vi "Autonomous Independent.vi"   [LabVIEW 2016]
doc: "This VI is called when autonomous begins, and will automatically be terminated when autonomous ends. You can carry out timed or sensor driven robot movement independently without needing to return to the caller."
uses:
  <vilib>/Rock Robotics/WPI/Solenoid/WPI_SolenoidValue.ctl
  <vilib>/Rock Robotics/WPI/Utilities/WPI_GetSetVariantRefNum.vi
  <vilib>/Rock Robotics/Network Tables/NT Read String.vi
  <vilib>/Rock Robotics/Network Tables/NT Write Numeric Array.vi
  Robot Global Data.vi
  <vilib>/Rock Robotics/WPI/Solenoid/WPI_SolenoidSetEnum.vi
  <vilib>/addons/control/pid/pid.llb/PID (DBL).vi
  <vilib>/addons/control/pid/NI_PID_pid.lvlib
panel:
  # "Be sure to right-click and choose Data Operations>>Make Current Value default if you want to save the array values with the VI"
types:
  T1 = typedef "WPI_JoystickDevRef.ctl" = cluster{"Device":T2}
  T2 = typedef "WPI_JoystickDeviceEnum.ctl" = enum16{"USB 0", "USB 1", "USB 2", "USB 3", "USB 4", "USB 5"}
  T3 = typedef "WPI_RobotDriveDevRef.ctl" = cluster{"DevStatus":errorcluster, "Motors[]":T4[], "Square Inputs":bool, "Max Output":dbl}
  T4 = typedef "WPI_MotorControlDeviceRef.ctl" = cluster{"DeviceStatus":errorcluster, "Type":T5, "PWM":cluster{"PWM Channel":T6, "DeadBand":T7}, "CAN":cluster{"Device Number":u8, "SetOutput VI Ref":variant, "GetOutput VI Ref":variant, "Enable VI Ref":variant, "Disable VI Ref":variant, "Data":variant}, "Invert":bool}
  T5 = typedef "WPI_MotorControlType.ctl" = enum16{"PWM", "CAN"}
  T6 = typedef "FPGA_DIOPWMChannel.ctl" = enum8{"PWM 0", "PWM 1", "PWM 2", "PWM 3", "PWM 4", "PWM 5", "PWM 6", "PWM 7", "PWM 8", "PWM 9", "PWM MXP 0", "PWM MXP 1", "PWM MXP 2", "PWM MXP 3", "PWM MXP 4", "PWM MXP 5", "PWM MXP 6", "PWM MXP 7", "PWM MXP 8", "PWM MXP 9", "Invalid"}
  T7 = typedef "WPI_PWMDeadband.ctl" = cluster{"Name":string, "maxPositivePwm":i32, "minPositivePwm":i32, "centerPwm":i32, "maxNegativePwm":i32, "minNegativePwm":i32, "angularRange":u16}
  T8 = typedef "WPI_EncoderDevRef.ctl" = cluster{"DevStatus":errorcluster, "EncoderIndex":T9, "CounterIndex":T10, "DistancePerCount":dbl, "Decoding Type":T11}
  T9 = typedef "FPGA_EncoderIdx.ctl" = enum8{"Enc 0", "Enc 1", "Enc 2", "Enc 3", "Enc 4", "Enc 5", "Enc 6", "Enc 7", "Invalid"}
  T10 = typedef "FPGA_CounterCtrSystemIndex.ctl" = enum8{"Ctr 0", "Ctr 1", "Ctr 2", "Ctr 3", "Ctr 4", "Ctr 5", "Ctr 6", "Ctr 7", "Invalid"}
  T11 = typedef "WPI_EncoderType.ctl" = enum16{"1x", "2x", "4x"}
  T12 = typedef "WPI_SolenoidDevRef.ctl" = cluster{"DevStatus":errorcluster, "Pneumatics Control Module":u8, "Forward Solenoid Channel":T13, "Reverse Solenoid Channel":T13}
  T13 = typedef "WPI_SolenoidChannel.ctl" = enum8{"Solenoid 0", "Solenoid 1", "Solenoid 2", "Solenoid 3", "Solenoid 4", "Solenoid 5", "Solenoid 6", "Solenoid 7", "Invalid"}
  T14 = typedef "WPI_SolenoidValue.ctl" = enum16{"Off", "On", "Forward", "Reverse"}
  T15 = cluster{"proportional gain (Kc)":dbl, "integral time (Ti, min)":dbl, "derivative time (Td, min)":dbl}
  T16 = cluster{"Yaw":dbl, "Roll":dbl, "Pitch":dbl, "Heading":dbl, "Fused Heading":dbl}
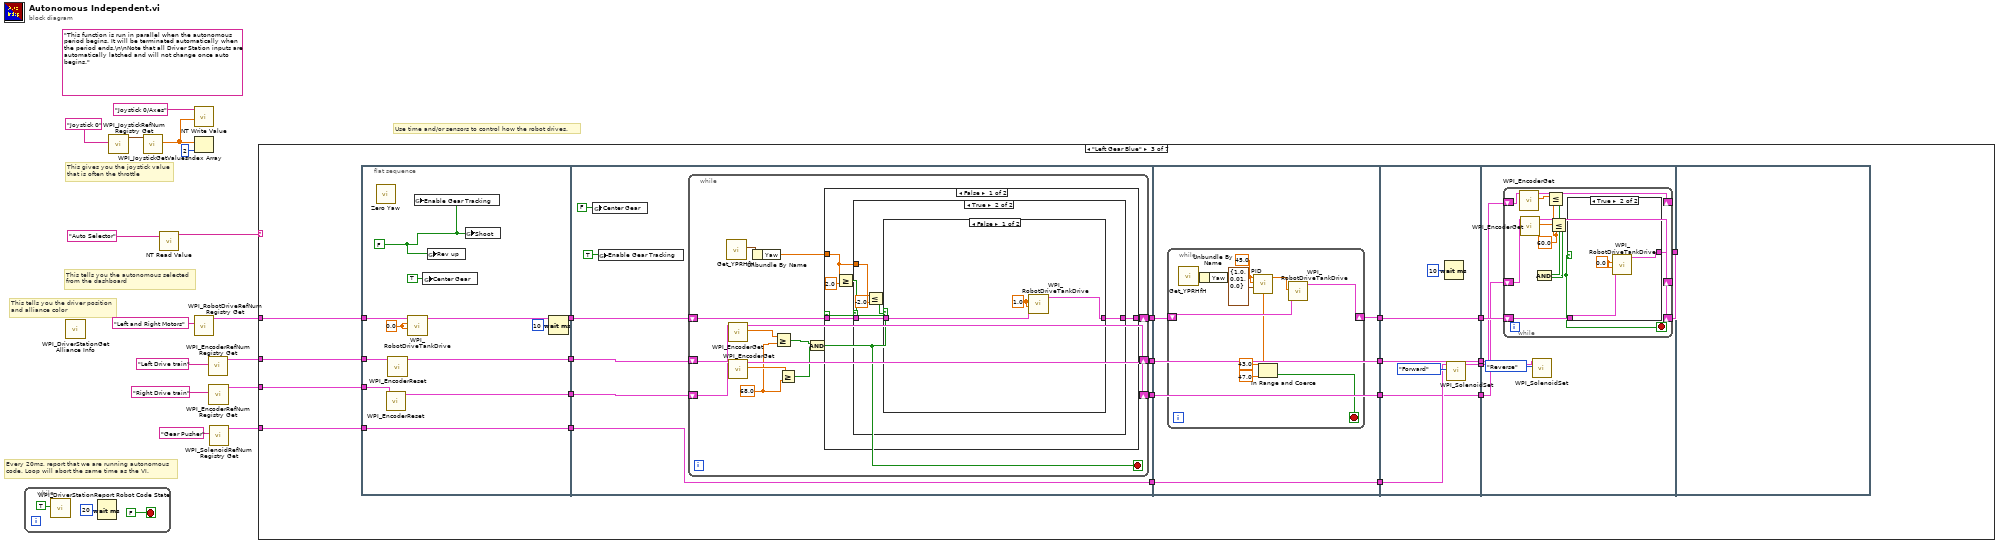
[diagram p0: block diagram]
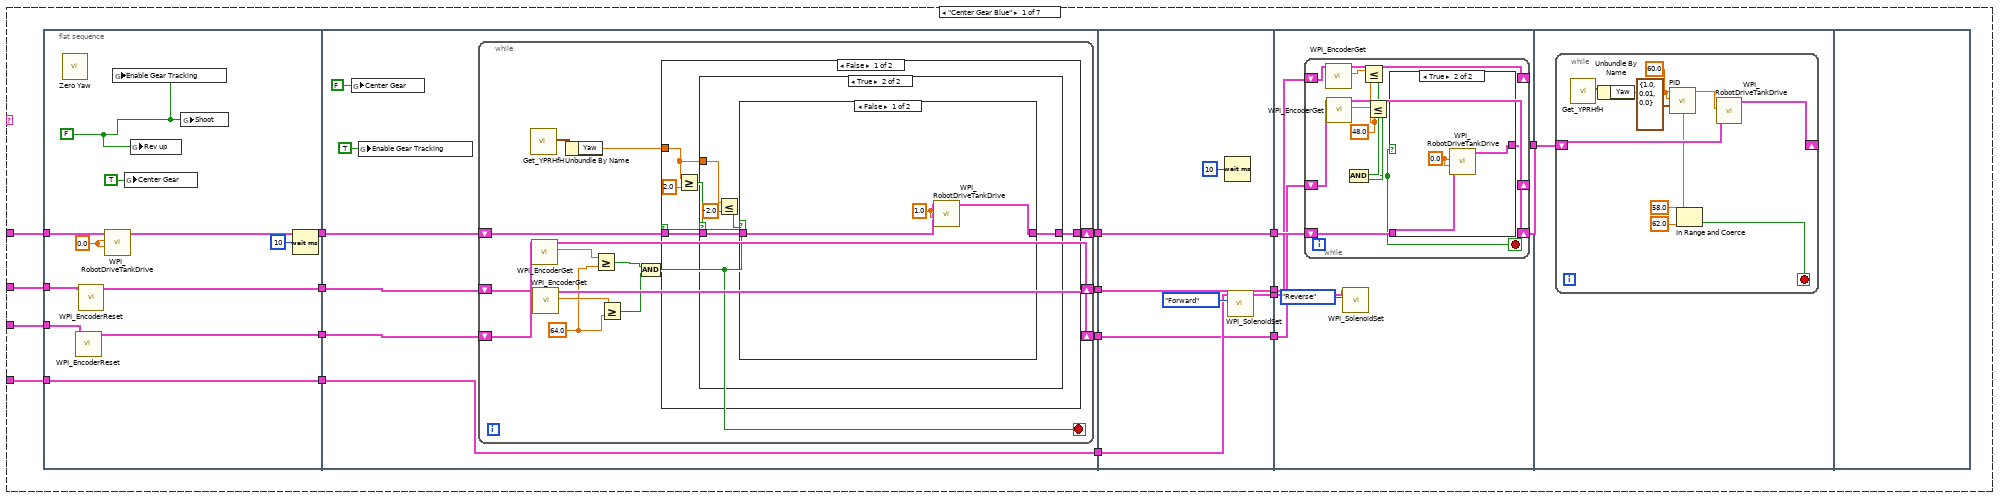
[diagram p2: hidden frame]
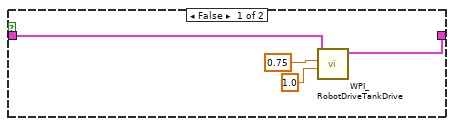
[diagram p3: hidden frame]
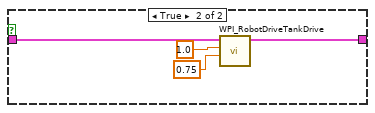
[diagram p4: hidden frame]
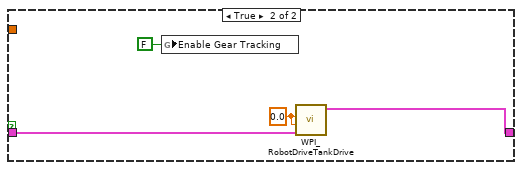
[diagram p5: hidden frame]
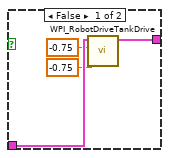
[diagram p6: hidden frame]
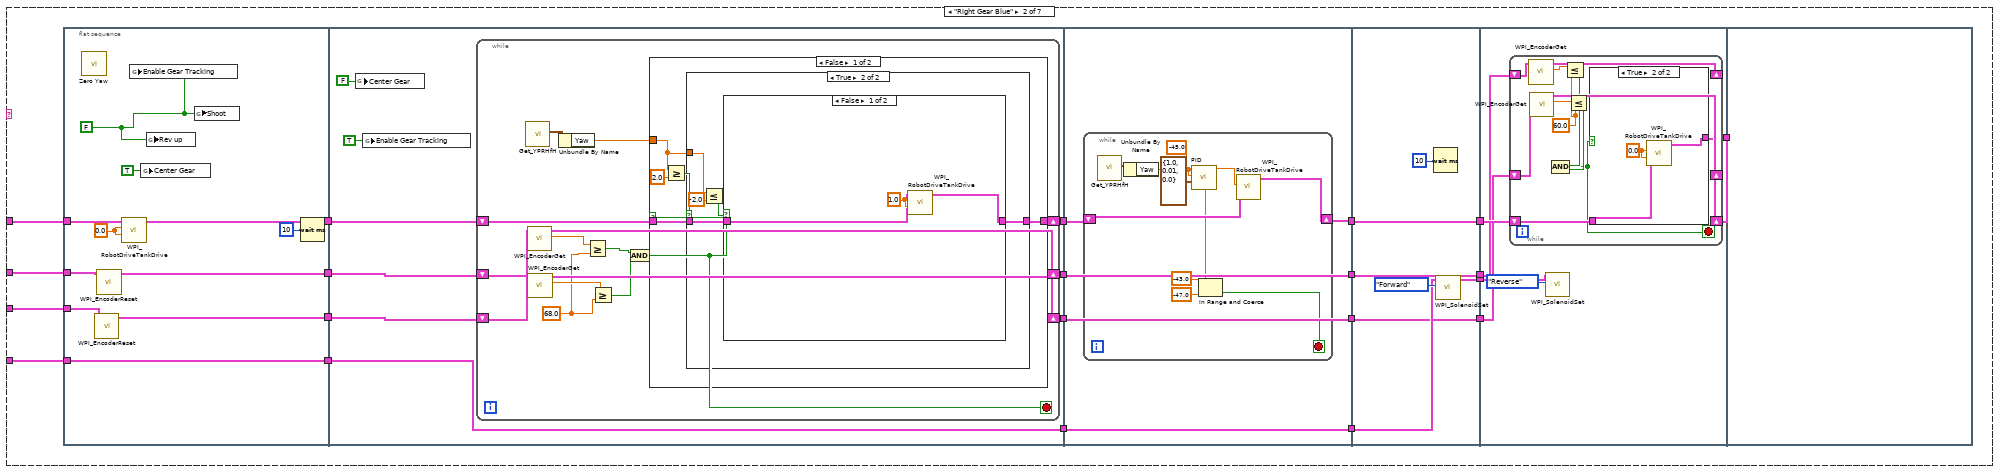
[diagram p7: hidden frame]
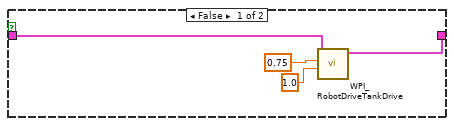
[diagram p8: hidden frame]
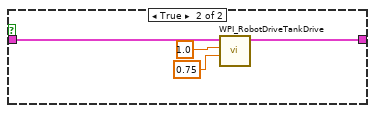
[diagram p9: hidden frame]
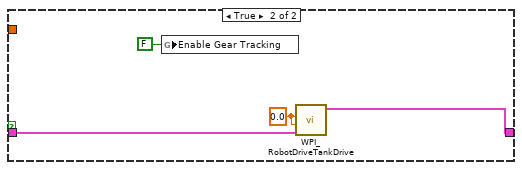
[diagram p10: hidden frame]
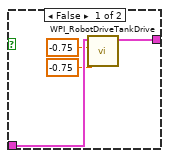
[diagram p11: hidden frame]
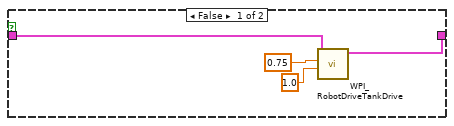
[diagram p12: hidden frame]
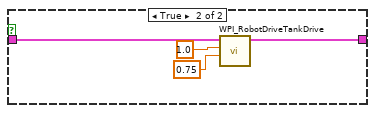
[diagram p13: hidden frame]
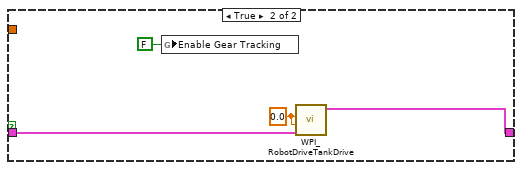
[diagram p14: hidden frame]
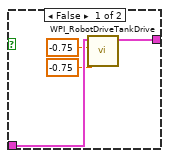
[diagram p15: hidden frame]
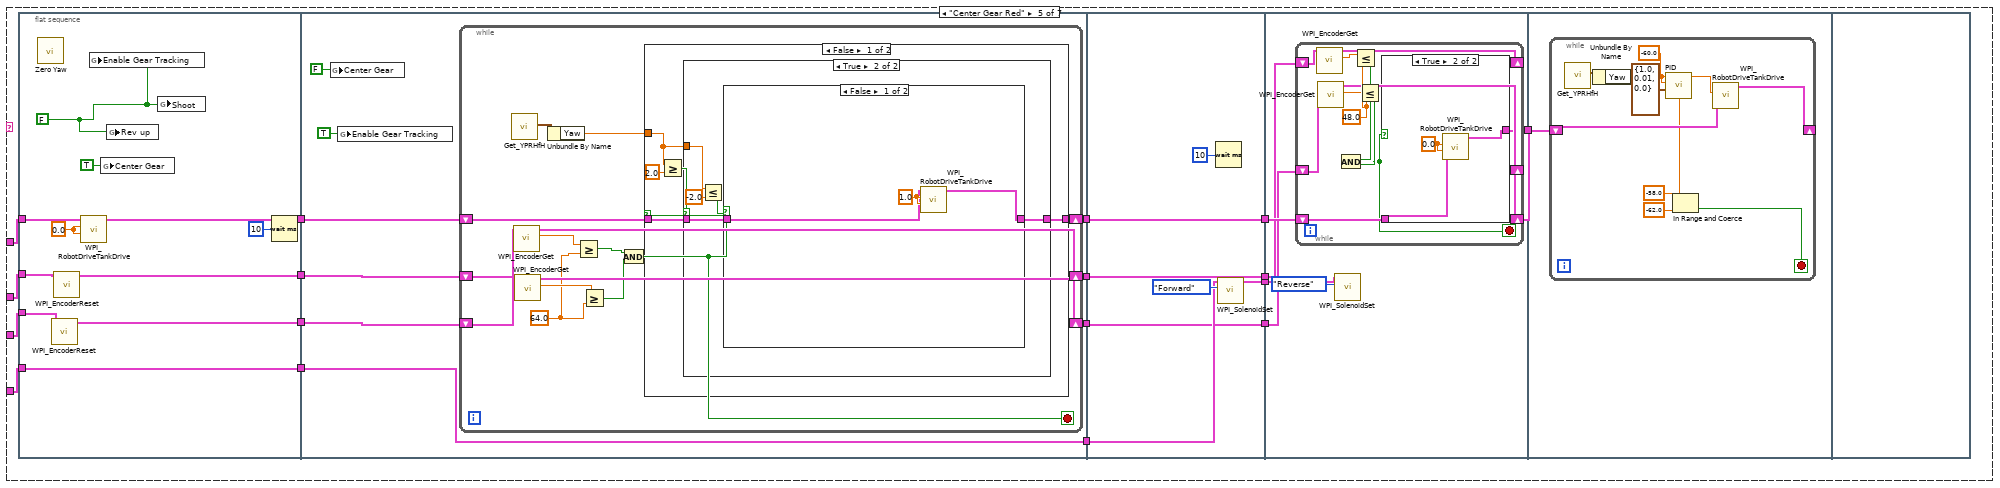
[diagram p17: hidden frame]
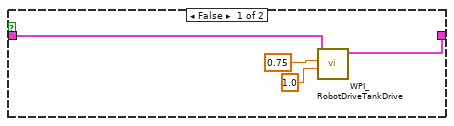
[diagram p18: hidden frame]
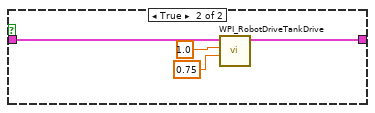
[diagram p19: hidden frame]
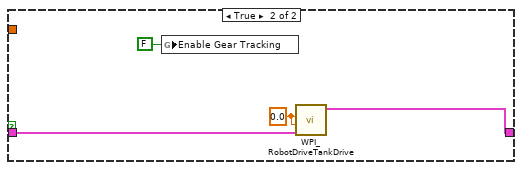
[diagram p20: hidden frame]
diagram:
  (unwired) "This function is run in parallel when the autonomous period begins. It will be terminated automatically when the period ends.\n\nNote that all Driver Station inputs are automatically latched and will not change once auto begins."
  # "This tells you the autonomous selected\nfrom the dashboard"
  # "Every 20ms, report that we are running autonomous\ncode. Loop will abort the same time as the VI."
  # "This gives you the joystick value\nthat is often the throttle"
  # "Use time and/or sensors to control how the robot drives."
  # "This tells you the driver position\nand alliance color"
  n1 = while {
    stop <- FALSE stop-if-true
    n2 = call <vilib>:"WPI_DriverStationReport Robot Code State.vi"("Autonomous"=TRUE) -> ()  [unwired: 10 in, 1 out]
    n3 = Wait (ms)(milliseconds to wait=u32 20) -> ()  [unwired: 1 out]
  }
  n4 = call <vilib>:"WPI_DriverStationGet Alliance Info.vi"() -> ()  [unwired: 12 out]
  n5 = call <vilib>:"WPI_JoystickRefNum Registry Get.vi"("refnum name"="Joystick 0") -> ("JoystickDevRef"=w14:T1)  [unwired: 1 in, 9 out]
  n6 = call <vilib>:"WPI_JoystickGetValues.vi"("JoystickDevRef"=w14) -> ("Axes"=w10:dbl[])  [unwired: 6 in, 4 out]
  n7 = call-poly <vilib>:"NT Read Value.vi"("Name"="Auto Selector") -> ("String"=w11:string)  [unwired: 9 in, 1 out]
  n8 = call-poly <vilib>:"NT Write Value.vi"("Numeric Array"=w10, "Name"="Joystick 0/Axes") -> ()  [unwired: 9 in, 1 out]
  n9 = Index Array(array=w10, index=2) -> ()  [unwired: 1 out]
  n10 = call <vilib>:"WPI_RobotDriveRefNum Registry Get.vi"("refnum name"="Left and Right Motors") -> ("RobotDriveDevRef"=w7:T3)  [unwired: 9 in, 1 out]
  n11 = call <vilib>:"WPI_EncoderRefNum Registry Get.vi"("refnum name"="Left Drive train") -> ("EncoderDevRef"=w4:T8)  [unwired: 9 in, 1 out]
  n12 = call <vilib>:"WPI_EncoderRefNum Registry Get.vi"("refnum name"="Right Drive train") -> ("EncoderDevRef"=w3:T8)  [unwired: 9 in, 1 out]
  n13 = call <vilib>:"WPI_SolenoidRefNum Registry Get.vi"("refnum name"="Gear Pusher") -> ("SolenoidDevRef"=w1:T12)  [unwired: 9 in, 1 out]
  n14 = case shown="\"Left Gear Blue\"" w11 {
    tunnel: w7 -> [w22 w138 w268 _ w408 w519 w641]
    tunnel: w4 -> [w21 w139 w267 _ w407 w520 w640]
    tunnel: w3 -> [w20 w140 w266 _ w406 w521 w639]
    tunnel: w1 -> [w19 w141 w265 _ w400 w522 w638]
    frame "Center Gear Blue" {
      n15 = flat-sequence {
        tunnel: w22 -> [w45]
        tunnel: w21 -> [w44]
        tunnel: w20 -> [w43]
        tunnel: [w39] -> w35
        tunnel: [w38] -> w34
        tunnel: [w37] -> w33
        tunnel: [w36] -> w32
        tunnel: w19 -> [w36]
        tunnel: w35 -> [w55]
        tunnel: w34 -> [w54]
        tunnel: w33 -> [w51]
        tunnel: [w50] -> w31
        tunnel: w32 -> [w50]
        tunnel: [w49] -> w30
        tunnel: [w48] -> w29
        tunnel: [w47] -> w28
        tunnel: w31 -> [w100]
        tunnel: [w98] -> w27
        tunnel: [w97] -> w26
        tunnel: w30 -> [w97]
        tunnel: [w96] -> w25
        tunnel: w29 -> [w96]
        tunnel: [w95] -> w24
        tunnel: w28 -> [w95]
        tunnel: w27 -> [w106]
        tunnel: w26 -> [w105]
        tunnel: w25 -> [w103]
        tunnel: w24 -> [w104]
        tunnel: [w102] -> w23
        tunnel: w23 -> [w127]
        frame #0 {
          w42 = FALSE
          w46 = 0.0 ("Left axis value")
          n16 = call <vilib>:"Zero Yaw.vi"() -> ()  [unwired: 12 in]
          n17 = call <vilib>:"WPI_EncoderReset.vi"("EncoderDevRef"=w43) -> ("EncoderDevRef"=w38:T8)  [unwired: 9 in, 1 out]
          n18 = call <vilib>:"WPI_EncoderReset.vi"("EncoderDevRef"=w44) -> ("EncoderDevRef"=w39:T8)  [unwired: 9 in, 1 out]
          n19 = call <vilib>:"WPI_RobotDriveTankDrive.vi"("Right axis value"=w46, "Left axis value"=w46, "RobotDriveDevRef"=w45) -> ("RobotDriveDevRef"=w37:T3)  [unwired: 6 in, 2 out]
          n20 = global write "Robot Global Data.vi" "Enable Gear Tracking"(w42) -> ()
          n21 = global write "Robot Global Data.vi" "Center Gear"(TRUE ("Center Gear")) -> ()
          n22 = global write "Robot Global Data.vi" "Rev up"(w42) -> ()
          n23 = global write "Robot Global Data.vi" "Shoot"(w42) -> ()
          n24 = Wait (ms)(milliseconds to wait=u32 10) -> ()  [unwired: 1 out]
        }
        frame #1 {
          n25 = global write "Robot Global Data.vi" "Center Gear"(FALSE ("Center Gear")) -> ()
          n26 = global write "Robot Global Data.vi" "Enable Gear Tracking"(TRUE ("Enable Gear Tracking")) -> ()
          n27 = while {
            shift-right: [w67] -> w48
            shift-left: w55 -> [w69]
            shift-right: [w66] -> w47
            shift-left: w54 -> [w68]
            shift-right: [w59] -> w49
            shift-left: w51 -> [w60]
            stop <- w63 stop-if-true
            w57 = 64.0
            n28 = call <vilib>:"Get_YPRHfH.vi"() -> ("YRPHfH"=w62:T16)  [unwired: 11 in]
            n29 = call <vilib>:"WPI_EncoderGet.vi"("EncoderDevRef"=w69) -> ("Distance"=w58:dbl, "EncoderDevRef"=w67:T8)  [unwired: 5 in, 4 out]
            n30 = call <vilib>:"WPI_EncoderGet.vi"("EncoderDevRef"=w68) -> ("Distance"=w65:dbl, "EncoderDevRef"=w66:T8)  [unwired: 5 in, 4 out]
            n31 = Unbundle By Name(w62) -> ("Yaw"=w61:dbl)
            n32 = Greater Or Equal?(x=w58, y=w57) -> (x >= y?=w56:bool)
            n33 = Greater Or Equal?(x=w65, y=w57) -> (x >= y?=w64:bool)
            n34 = Compound Arithmetic op=AND(w56, w64) -> (w63:bool)
            n35 = case shown="False" w63 {
              tunnel: w61 -> [w72 _]
              tunnel: w60 -> [w71 w93]
              tunnel: [w70 w92] -> w59
              frame False {
                n36 = Greater Or Equal?(x=w72, y=2.0) -> (x >= y?=w73:bool)
                n37 = case shown="True" w73 {
                  tunnel: w72 -> [_ w83]
                  tunnel: w71 -> [w76 w80]
                  tunnel: [w75 w79] -> w70
                  frame False {
                    n38 = call <vilib>:"WPI_RobotDriveTankDrive.vi"("Right axis value"=1.0, "Left axis value"=0.75, "RobotDriveDevRef"=w76) -> ("RobotDriveDevRef"=w75:T3)  [unwired: 6 in, 2 out]
                  }
                  frame True {
                    n39 = Less Or Equal?(x=w83, y=-2.0) -> (x <= y?=w81:bool)
                    n40 = case shown="False" w81 {
                      tunnel: w80 -> [w85 w88]
                      tunnel: [w84 w87] -> w79
                      frame False {
                        w86 = 1.0 ("Left axis value")
                        n41 = call <vilib>:"WPI_RobotDriveTankDrive.vi"("Right axis value"=w86, "Left axis value"=w86, "RobotDriveDevRef"=w85) -> ("RobotDriveDevRef"=w84:T3)  [unwired: 6 in, 2 out]
                      }
                      frame True {
                        n42 = call <vilib>:"WPI_RobotDriveTankDrive.vi"("Right axis value"=0.75, "Left axis value"=1.0, "RobotDriveDevRef"=w88) -> ("RobotDriveDevRef"=w87:T3)  [unwired: 6 in, 2 out]
                      }
                    }
                  }
                }
              }
              frame True {
                w94 = 0.0 ("Left axis value")
                n43 = global write "Robot Global Data.vi" "Enable Gear Tracking"(FALSE ("Enable Gear Tracking")) -> ()
                n44 = call <vilib>:"WPI_RobotDriveTankDrive.vi"("Right axis value"=w94, "Left axis value"=w94, "RobotDriveDevRef"=w93) -> ("RobotDriveDevRef"=w92:T3)  [unwired: 6 in, 2 out]
              }
            }
          }
        }
        frame #2 {
          n45 = Wait (ms)(milliseconds to wait=u32 10) -> ()  [unwired: 1 out]
          n46 = call-poly <vilib>:"WPI_SolenoidSet.vi"("Value"=WPI_SolenoidValue."Forward", "SolenoidDevRef"=w100) -> ("SolenoidDevRef"=w98:T12)  [unwired: 8 in, 1 out]
        }
        frame #3 {
          n47 = while {
            shift-right: [w112] -> _
            shift-left: w104 -> [w114]
            shift-right: [w113] -> _
            shift-left: w103 -> [w115]
            shift-right: [w108] -> w102
            shift-left: w105 -> [w119]
            stop <- w109 stop-if-true
            w117 = 48.0
            n48 = call <vilib>:"WPI_EncoderGet.vi"("EncoderDevRef"=w115) -> ("Distance"=w118:dbl, "EncoderDevRef"=w113:T8)  [unwired: 5 in, 4 out]
            n49 = call <vilib>:"WPI_EncoderGet.vi"("EncoderDevRef"=w114) -> ("Distance"=w116:dbl, "EncoderDevRef"=w112:T8)  [unwired: 5 in, 4 out]
            n50 = Less Or Equal?(x=w118, y=w117) -> (x <= y?=w111:bool)
            n51 = Less Or Equal?(x=w116, y=w117) -> (x <= y?=w110:bool)
            n52 = Compound Arithmetic op=AND(w111, w110) -> (w109:bool)
            n53 = case shown="True" w109 {
              tunnel: w119 -> [w123 w125]
              tunnel: [w120 w124] -> w108
              frame False {
                n54 = call <vilib>:"WPI_RobotDriveTankDrive.vi"("Right axis value"=-0.75, "Left axis value"=-0.75, "RobotDriveDevRef"=w123) -> ("RobotDriveDevRef"=w120:T3)  [unwired: 6 in, 2 out]
              }
              frame True {
                w126 = 0.0 ("Left axis value")
                n55 = call <vilib>:"WPI_RobotDriveTankDrive.vi"("Right axis value"=w126, "Left axis value"=w126, "RobotDriveDevRef"=w125) -> ("RobotDriveDevRef"=w124:T3)  [unwired: 6 in, 2 out]
              }
            }
          }
          n56 = call-poly <vilib>:"WPI_SolenoidSet.vi"("Value"=WPI_SolenoidValue."Reverse", "SolenoidDevRef"=w106) -> ()  [unwired: 8 in, 2 out]
        }
        frame #4 {
          n57 = while {
            shift-right: [w132] -> _
            shift-left: w127 -> [w133]
            stop <- w128 stop-if-true
            n58 = call <vilib>:"Get_YPRHfH.vi"() -> ("YRPHfH"=w137:T16)  [unwired: 11 in]
            n59 = Unbundle By Name(w137) -> ("Yaw"=w131:dbl)
            n60 = call-poly <vilib>:"PID.vi"("PID gains"=T15 {"proportional gain (Kc)"=1.0, "integral time (Ti, min)"=0.01, "derivative time (Td, min)"=0.0}, "process variable"=w131, "setpoint"=60.0) -> ("output"=w134:dbl)  [unwired: 7 in, 1 out]
            n61 = In Range and Coerce(upper limit=58.0, x=w131, lower limit=62.0) -> (In Range?=w128:bool)  [unwired: 1 out]
            n62 = call <vilib>:"WPI_RobotDriveTankDrive.vi"("Left axis value"=w134, "RobotDriveDevRef"=w133) -> ("RobotDriveDevRef"=w132:T3)  [unwired: 7 in, 2 out]
          }
        }
        frame #5 {
        }
      }
    }
    frame "Right Gear Blue" {
      n63 = flat-sequence {
        tunnel: w138 -> [w168]
        tunnel: w139 -> [w167]
        tunnel: [w163] -> w158
        tunnel: [w162] -> w157
        tunnel: [w161] -> w156
        tunnel: [w160] -> w155
        tunnel: w141 -> [w160]
        tunnel: w140 -> [w159]
        tunnel: w158 -> [w178]
        tunnel: w157 -> [w177]
        tunnel: w156 -> [w174]
        tunnel: [w173] -> w154
        tunnel: w155 -> [w173]
        tunnel: [w172] -> w153
        tunnel: [w171] -> w152
        tunnel: [w170] -> w151
        tunnel: w154 -> [w222]
        tunnel: [w222] -> w150
        tunnel: w153 -> [w221]
        tunnel: [w220] -> w149
        tunnel: w152 -> [w219]
        tunnel: [w219] -> w148
        tunnel: w151 -> [w218]
        tunnel: [w218] -> w147
        tunnel: w150 -> [w238]
        tunnel: [w236] -> w146
        tunnel: [w235] -> w145
        tunnel: w149 -> [w235]
        tunnel: [w234] -> w144
        tunnel: w148 -> [w234]
        tunnel: [w233] -> w143
        tunnel: w147 -> [w233]
        tunnel: w146 -> [w244]
        tunnel: w145 -> [w243]
        tunnel: w144 -> [w241]
        tunnel: w143 -> [w242]
        tunnel: [w240] -> w142
        tunnel: w142 -> [_]
        frame #0 {
          w166 = FALSE
          w169 = 0.0 ("Left axis value")
          n64 = call <vilib>:"Zero Yaw.vi"() -> ()  [unwired: 12 in]
          n65 = call <vilib>:"WPI_EncoderReset.vi"("EncoderDevRef"=w159) -> ("EncoderDevRef"=w162:T8)  [unwired: 9 in, 1 out]
          n66 = call <vilib>:"WPI_EncoderReset.vi"("EncoderDevRef"=w167) -> ("EncoderDevRef"=w163:T8)  [unwired: 9 in, 1 out]
          n67 = call <vilib>:"WPI_RobotDriveTankDrive.vi"("Right axis value"=w169, "Left axis value"=w169, "RobotDriveDevRef"=w168) -> ("RobotDriveDevRef"=w161:T3)  [unwired: 6 in, 2 out]
          n68 = global write "Robot Global Data.vi" "Enable Gear Tracking"(w166) -> ()
          n69 = global write "Robot Global Data.vi" "Center Gear"(TRUE ("Center Gear")) -> ()
          n70 = global write "Robot Global Data.vi" "Rev up"(w166) -> ()
          n71 = global write "Robot Global Data.vi" "Shoot"(w166) -> ()
          n72 = Wait (ms)(milliseconds to wait=u32 10) -> ()  [unwired: 1 out]
        }
        frame #1 {
          n73 = global write "Robot Global Data.vi" "Center Gear"(FALSE ("Center Gear")) -> ()
          n74 = global write "Robot Global Data.vi" "Enable Gear Tracking"(TRUE ("Enable Gear Tracking")) -> ()
          n75 = while {
            shift-right: [w190] -> w171
            shift-left: w178 -> [w192]
            shift-right: [w189] -> w170
            shift-left: w177 -> [w191]
            shift-right: [w182] -> w172
            shift-left: w174 -> [w183]
            stop <- w186 stop-if-true
            w180 = 68.0
            n76 = call <vilib>:"Get_YPRHfH.vi"() -> ("YRPHfH"=w185:T16)  [unwired: 11 in]
            n77 = call <vilib>:"WPI_EncoderGet.vi"("EncoderDevRef"=w192) -> ("Distance"=w181:dbl, "EncoderDevRef"=w190:T8)  [unwired: 5 in, 4 out]
            n78 = call <vilib>:"WPI_EncoderGet.vi"("EncoderDevRef"=w191) -> ("Distance"=w188:dbl, "EncoderDevRef"=w189:T8)  [unwired: 5 in, 4 out]
            n79 = Unbundle By Name(w185) -> ("Yaw"=w184:dbl)
            n80 = Greater Or Equal?(x=w181, y=w180) -> (x >= y?=w179:bool)
            n81 = Greater Or Equal?(x=w188, y=w180) -> (x >= y?=w187:bool)
            n82 = Compound Arithmetic op=AND(w179, w187) -> (w186:bool)
            n83 = case shown="False" w186 {
              tunnel: w184 -> [w195 _]
              tunnel: w183 -> [w194 w216]
              tunnel: [w193 w215] -> w182
              frame False {
                n84 = Greater Or Equal?(x=w195, y=2.0) -> (x >= y?=w196:bool)
                n85 = case shown="True" w196 {
                  tunnel: w195 -> [_ w206]
                  tunnel: w194 -> [w199 w203]
                  tunnel: [w198 w202] -> w193
                  frame False {
                    n86 = call <vilib>:"WPI_RobotDriveTankDrive.vi"("Right axis value"=1.0, "Left axis value"=0.75, "RobotDriveDevRef"=w199) -> ("RobotDriveDevRef"=w198:T3)  [unwired: 6 in, 2 out]
                  }
                  frame True {
                    n87 = Less Or Equal?(x=w206, y=-2.0) -> (x <= y?=w204:bool)
                    n88 = case shown="False" w204 {
                      tunnel: w203 -> [w208 w211]
                      tunnel: [w207 w210] -> w202
                      frame False {
                        w209 = 1.0 ("Left axis value")
                        n89 = call <vilib>:"WPI_RobotDriveTankDrive.vi"("Right axis value"=w209, "Left axis value"=w209, "RobotDriveDevRef"=w208) -> ("RobotDriveDevRef"=w207:T3)  [unwired: 6 in, 2 out]
                      }
                      frame True {
                        n90 = call <vilib>:"WPI_RobotDriveTankDrive.vi"("Right axis value"=0.75, "Left axis value"=1.0, "RobotDriveDevRef"=w211) -> ("RobotDriveDevRef"=w210:T3)  [unwired: 6 in, 2 out]
                      }
                    }
                  }
                }
              }
              frame True {
                w217 = 0.0 ("Left axis value")
                n91 = global write "Robot Global Data.vi" "Enable Gear Tracking"(FALSE ("Enable Gear Tracking")) -> ()
                n92 = call <vilib>:"WPI_RobotDriveTankDrive.vi"("Right axis value"=w217, "Left axis value"=w217, "RobotDriveDevRef"=w216) -> ("RobotDriveDevRef"=w215:T3)  [unwired: 6 in, 2 out]
              }
            }
          }
        }
        frame #2 {
          n93 = while {
            shift-right: [w227] -> w220
            shift-left: w221 -> [w228]
            stop <- w223 stop-if-true
            n94 = call <vilib>:"Get_YPRHfH.vi"() -> ("YRPHfH"=w232:T16)  [unwired: 11 in]
            n95 = Unbundle By Name(w232) -> ("Yaw"=w226:dbl)
            n96 = call-poly <vilib>:"PID.vi"("PID gains"=T15 {"proportional gain (Kc)"=1.0, "integral time (Ti, min)"=0.01, "derivative time (Td, min)"=0.0}, "process variable"=w226, "setpoint"=-45.0) -> ("output"=w229:dbl)  [unwired: 7 in, 1 out]
            n97 = In Range and Coerce(upper limit=-43.0, x=w226, lower limit=-47.0) -> (In Range?=w223:bool)  [unwired: 1 out]
            n98 = call <vilib>:"WPI_RobotDriveTankDrive.vi"("Left axis value"=w229, "RobotDriveDevRef"=w228) -> ("RobotDriveDevRef"=w227:T3)  [unwired: 7 in, 2 out]
          }
        }
        frame #3 {
          n99 = Wait (ms)(milliseconds to wait=u32 10) -> ()  [unwired: 1 out]
          n100 = call-poly <vilib>:"WPI_SolenoidSet.vi"("Value"=WPI_SolenoidValue."Forward", "SolenoidDevRef"=w238) -> ("SolenoidDevRef"=w236:T12)  [unwired: 8 in, 1 out]
        }
        frame #4 {
          n101 = while {
            shift-right: [w250] -> _
            shift-left: w242 -> [w252]
            shift-right: [w251] -> _
            shift-left: w241 -> [w253]
            shift-right: [w246] -> w240
            shift-left: w243 -> [w257]
            stop <- w247 stop-if-true
            w255 = 60.0
            n102 = call <vilib>:"WPI_EncoderGet.vi"("EncoderDevRef"=w253) -> ("Distance"=w256:dbl, "EncoderDevRef"=w251:T8)  [unwired: 5 in, 4 out]
            n103 = call <vilib>:"WPI_EncoderGet.vi"("EncoderDevRef"=w252) -> ("Distance"=w254:dbl, "EncoderDevRef"=w250:T8)  [unwired: 5 in, 4 out]
            n104 = Less Or Equal?(x=w256, y=w255) -> (x <= y?=w249:bool)
            n105 = Less Or Equal?(x=w254, y=w255) -> (x <= y?=w248:bool)
            n106 = Compound Arithmetic op=AND(w249, w248) -> (w247:bool)
            n107 = case shown="True" w247 {
              tunnel: w257 -> [w261 w263]
              tunnel: [w258 w262] -> w246
              frame False {
                n108 = call <vilib>:"WPI_RobotDriveTankDrive.vi"("Right axis value"=-0.75, "Left axis value"=-0.75, "RobotDriveDevRef"=w261) -> ("RobotDriveDevRef"=w258:T3)  [unwired: 6 in, 2 out]
              }
              frame True {
                w264 = 0.0 ("Left axis value")
                n109 = call <vilib>:"WPI_RobotDriveTankDrive.vi"("Right axis value"=w264, "Left axis value"=w264, "RobotDriveDevRef"=w263) -> ("RobotDriveDevRef"=w262:T3)  [unwired: 6 in, 2 out]
              }
            }
          }
          n110 = call-poly <vilib>:"WPI_SolenoidSet.vi"("Value"=WPI_SolenoidValue."Reverse", "SolenoidDevRef"=w244) -> ()  [unwired: 8 in, 2 out]
        }
        frame #5 {
        }
      }
    }
    frame "Left Gear Blue" {
      n111 = flat-sequence {
        tunnel: w268 -> [w295]
        tunnel: w267 -> [w294]
        tunnel: w266 -> [w293]
        tunnel: [w289] -> w285
        tunnel: [w288] -> w284
        tunnel: [w287] -> w283
        tunnel: [w286] -> w282
        tunnel: w265 -> [w286]
        tunnel: w285 -> [w305]
        tunnel: w284 -> [w304]
        tunnel: w283 -> [w301]
        tunnel: [w300] -> w281
        tunnel: w282 -> [w300]
        tunnel: [w299] -> w280
        tunnel: [w298] -> w279
        tunnel: [w297] -> w278
        tunnel: w281 -> [w349]
        tunnel: [w349] -> w277
        tunnel: w280 -> [w348]
        tunnel: [w347] -> w276
        tunnel: w279 -> [w346]
        tunnel: [w346] -> w275
        tunnel: w278 -> [w345]
        tunnel: [w345] -> w274
        tunnel: w277 -> [w365]
        tunnel: [w363] -> w273
        tunnel: [w362] -> w272
        tunnel: w276 -> [w362]
        tunnel: [w361] -> w271
        tunnel: w275 -> [w361]
        tunnel: [w360] -> w270
        tunnel: w274 -> [w360]
        tunnel: w273 -> [w371]
        tunnel: w272 -> [w370]
        tunnel: w271 -> [w368]
        tunnel: w270 -> [w369]
        tunnel: [w367] -> w269
        tunnel: w269 -> [_]
        frame #0 {
          w292 = FALSE
          w296 = 0.0 ("Left axis value")
          n112 = call <vilib>:"Zero Yaw.vi"() -> ()  [unwired: 12 in]
          n113 = call <vilib>:"WPI_EncoderReset.vi"("EncoderDevRef"=w293) -> ("EncoderDevRef"=w288:T8)  [unwired: 9 in, 1 out]
          n114 = call <vilib>:"WPI_EncoderReset.vi"("EncoderDevRef"=w294) -> ("EncoderDevRef"=w289:T8)  [unwired: 9 in, 1 out]
          n115 = call <vilib>:"WPI_RobotDriveTankDrive.vi"("Right axis value"=w296, "Left axis value"=w296, "RobotDriveDevRef"=w295) -> ("RobotDriveDevRef"=w287:T3)  [unwired: 6 in, 2 out]
          n116 = global write "Robot Global Data.vi" "Enable Gear Tracking"(w292) -> ()
          n117 = global write "Robot Global Data.vi" "Center Gear"(TRUE ("Center Gear")) -> ()
          n118 = global write "Robot Global Data.vi" "Rev up"(w292) -> ()
          n119 = global write "Robot Global Data.vi" "Shoot"(w292) -> ()
          n120 = Wait (ms)(milliseconds to wait=u32 10) -> ()  [unwired: 1 out]
        }
        frame #1 {
          n121 = global write "Robot Global Data.vi" "Center Gear"(FALSE ("Center Gear")) -> ()
          n122 = global write "Robot Global Data.vi" "Enable Gear Tracking"(TRUE ("Enable Gear Tracking")) -> ()
          n123 = while {
            shift-right: [w317] -> w298
            shift-left: w305 -> [w319]
            shift-right: [w316] -> w297
            shift-left: w304 -> [w318]
            shift-right: [w309] -> w299
            shift-left: w301 -> [w310]
            stop <- w313 stop-if-true
            w307 = 68.0
            n124 = call <vilib>:"Get_YPRHfH.vi"() -> ("YRPHfH"=w312:T16)  [unwired: 11 in]
            n125 = call <vilib>:"WPI_EncoderGet.vi"("EncoderDevRef"=w319) -> ("Distance"=w308:dbl, "EncoderDevRef"=w317:T8)  [unwired: 5 in, 4 out]
            n126 = call <vilib>:"WPI_EncoderGet.vi"("EncoderDevRef"=w318) -> ("Distance"=w315:dbl, "EncoderDevRef"=w316:T8)  [unwired: 5 in, 4 out]
            n127 = Unbundle By Name(w312) -> ("Yaw"=w311:dbl)
            n128 = Greater Or Equal?(x=w308, y=w307) -> (x >= y?=w306:bool)
            n129 = Greater Or Equal?(x=w315, y=w307) -> (x >= y?=w314:bool)
            n130 = Compound Arithmetic op=AND(w306, w314) -> (w313:bool)
            n131 = case shown="False" w313 {
              tunnel: w311 -> [w322 _]
              tunnel: w310 -> [w321 w343]
              tunnel: [w320 w342] -> w309
              frame False {
                n132 = Greater Or Equal?(x=w322, y=2.0) -> (x >= y?=w323:bool)
                n133 = case shown="True" w323 {
                  tunnel: w322 -> [_ w333]
                  tunnel: w321 -> [w326 w330]
                  tunnel: [w325 w329] -> w320
                  frame False {
                    n134 = call <vilib>:"WPI_RobotDriveTankDrive.vi"("Right axis value"=1.0, "Left axis value"=0.75, "RobotDriveDevRef"=w326) -> ("RobotDriveDevRef"=w325:T3)  [unwired: 6 in, 2 out]
                  }
                  frame True {
                    n135 = Less Or Equal?(x=w333, y=-2.0) -> (x <= y?=w331:bool)
                    n136 = case shown="False" w331 {
                      tunnel: w330 -> [w335 w338]
                      tunnel: [w334 w337] -> w329
                      frame False {
                        w336 = 1.0 ("Left axis value")
                        n137 = call <vilib>:"WPI_RobotDriveTankDrive.vi"("Right axis value"=w336, "Left axis value"=w336, "RobotDriveDevRef"=w335) -> ("RobotDriveDevRef"=w334:T3)  [unwired: 6 in, 2 out]
                      }
                      frame True {
                        n138 = call <vilib>:"WPI_RobotDriveTankDrive.vi"("Right axis value"=0.75, "Left axis value"=1.0, "RobotDriveDevRef"=w338) -> ("RobotDriveDevRef"=w337:T3)  [unwired: 6 in, 2 out]
                      }
                    }
                  }
                }
              }
              frame True {
                w344 = 0.0 ("Left axis value")
                n139 = global write "Robot Global Data.vi" "Enable Gear Tracking"(FALSE ("Enable Gear Tracking")) -> ()
                n140 = call <vilib>:"WPI_RobotDriveTankDrive.vi"("Right axis value"=w344, "Left axis value"=w344, "RobotDriveDevRef"=w343) -> ("RobotDriveDevRef"=w342:T3)  [unwired: 6 in, 2 out]
              }
            }
          }
        }
        frame #2 {
          n141 = while {
            shift-right: [w354] -> w347
            shift-left: w348 -> [w355]
            stop <- w350 stop-if-true
            n142 = call <vilib>:"Get_YPRHfH.vi"() -> ("YRPHfH"=w359:T16)  [unwired: 11 in]
            n143 = Unbundle By Name(w359) -> ("Yaw"=w353:dbl)
            n144 = call-poly <vilib>:"PID.vi"("PID gains"=T15 {"proportional gain (Kc)"=1.0, "integral time (Ti, min)"=0.01, "derivative time (Td, min)"=0.0}, "process variable"=w353, "setpoint"=45.0) -> ("output"=w356:dbl)  [unwired: 7 in, 1 out]
            n145 = In Range and Coerce(upper limit=43.0, x=w353, lower limit=47.0) -> (In Range?=w350:bool)  [unwired: 1 out]
            n146 = call <vilib>:"WPI_RobotDriveTankDrive.vi"("Left axis value"=w356, "RobotDriveDevRef"=w355) -> ("RobotDriveDevRef"=w354:T3)  [unwired: 7 in, 2 out]
          }
        }
        frame #3 {
          n147 = Wait (ms)(milliseconds to wait=u32 10) -> ()  [unwired: 1 out]
          n148 = call-poly <vilib>:"WPI_SolenoidSet.vi"("Value"=WPI_SolenoidValue."Forward", "SolenoidDevRef"=w365) -> ("SolenoidDevRef"=w363:T12)  [unwired: 8 in, 1 out]
        }
        frame #4 {
          n149 = while {
            shift-right: [w377] -> _
            shift-left: w369 -> [w379]
            shift-right: [w378] -> _
            shift-left: w368 -> [w380]
            shift-right: [w373] -> w367
            shift-left: w370 -> [w384]
            stop <- w374 stop-if-true
            w382 = 60.0
            n150 = call <vilib>:"WPI_EncoderGet.vi"("EncoderDevRef"=w380) -> ("Distance"=w383:dbl, "EncoderDevRef"=w378:T8)  [unwired: 5 in, 4 out]
            n151 = call <vilib>:"WPI_EncoderGet.vi"("EncoderDevRef"=w379) -> ("Distance"=w381:dbl, "EncoderDevRef"=w377:T8)  [unwired: 5 in, 4 out]
            n152 = Less Or Equal?(x=w383, y=w382) -> (x <= y?=w376:bool)
            n153 = Less Or Equal?(x=w381, y=w382) -> (x <= y?=w375:bool)
            n154 = Compound Arithmetic op=AND(w376, w375) -> (w374:bool)
            n155 = case shown="True" w374 {
              tunnel: w384 -> [w388 w390]
              tunnel: [w385 w389] -> w373
              frame False {
                n156 = call <vilib>:"WPI_RobotDriveTankDrive.vi"("Right axis value"=-0.75, "Left axis value"=-0.75, "RobotDriveDevRef"=w388) -> ("RobotDriveDevRef"=w385:T3)  [unwired: 6 in, 2 out]
              }
              frame True {
                w391 = 0.0 ("Left axis value")
                n157 = call <vilib>:"WPI_RobotDriveTankDrive.vi"("Right axis value"=w391, "Left axis value"=w391, "RobotDriveDevRef"=w390) -> ("RobotDriveDevRef"=w389:T3)  [unwired: 6 in, 2 out]
              }
            }
          }
          n158 = call-poly <vilib>:"WPI_SolenoidSet.vi"("Value"=WPI_SolenoidValue."Reverse", "SolenoidDevRef"=w371) -> ()  [unwired: 8 in, 2 out]
        }
        frame #5 {
        }
      }
    }
    frame Default {
    }
    frame "Center Gear Red" {
      n159 = flat-sequence {
        tunnel: w408 -> [w418]
        tunnel: w407 -> [w417]
        tunnel: w406 -> [w416]
        tunnel: [w412] -> w405
        tunnel: [w411] -> w404
        tunnel: [w410] -> w403
        tunnel: [w409] -> w401
        tunnel: w400 -> [w409]
        tunnel: w405 -> [w428]
        tunnel: w404 -> [w427]
        tunnel: w403 -> [w424]
        tunnel: [w423] -> w402
        tunnel: w401 -> [w423]
        tunnel: [w422] -> w397
        tunnel: [w421] -> w395
        tunnel: [w420] -> w393
        tunnel: w402 -> [w473]
        tunnel: [w471] -> w399
        tunnel: [w470] -> w398
        tunnel: w397 -> [w470]
        tunnel: [w469] -> w396
        tunnel: w395 -> [w469]
        tunnel: [w468] -> w394
        tunnel: w393 -> [w468]
        tunnel: w399 -> [w479]
        tunnel: w398 -> [w478]
        tunnel: w396 -> [w476]
        tunnel: w394 -> [w477]
        tunnel: [w475] -> w392
        tunnel: w392 -> [w500]
        frame #0 {
          w415 = FALSE
          w419 = 0.0 ("Left axis value")
          n160 = call <vilib>:"Zero Yaw.vi"() -> ()  [unwired: 12 in]
          n161 = call <vilib>:"WPI_EncoderReset.vi"("EncoderDevRef"=w416) -> ("EncoderDevRef"=w411:T8)  [unwired: 9 in, 1 out]
          n162 = call <vilib>:"WPI_EncoderReset.vi"("EncoderDevRef"=w417) -> ("EncoderDevRef"=w412:T8)  [unwired: 9 in, 1 out]
          n163 = call <vilib>:"WPI_RobotDriveTankDrive.vi"("Right axis value"=w419, "Left axis value"=w419, "RobotDriveDevRef"=w418) -> ("RobotDriveDevRef"=w410:T3)  [unwired: 6 in, 2 out]
          n164 = global write "Robot Global Data.vi" "Enable Gear Tracking"(w415) -> ()
          n165 = global write "Robot Global Data.vi" "Center Gear"(TRUE ("Center Gear")) -> ()
          n166 = global write "Robot Global Data.vi" "Rev up"(w415) -> ()
          n167 = global write "Robot Global Data.vi" "Shoot"(w415) -> ()
          n168 = Wait (ms)(milliseconds to wait=u32 10) -> ()  [unwired: 1 out]
        }
        frame #1 {
          n169 = global write "Robot Global Data.vi" "Center Gear"(FALSE ("Center Gear")) -> ()
          n170 = global write "Robot Global Data.vi" "Enable Gear Tracking"(TRUE ("Enable Gear Tracking")) -> ()
          n171 = while {
            shift-right: [w440] -> w421
            shift-left: w428 -> [w442]
            shift-right: [w439] -> w420
            shift-left: w427 -> [w441]
            shift-right: [w432] -> w422
            shift-left: w424 -> [w433]
            stop <- w436 stop-if-true
            w430 = 64.0
            n172 = call <vilib>:"Get_YPRHfH.vi"() -> ("YRPHfH"=w435:T16)  [unwired: 11 in]
            n173 = call <vilib>:"WPI_EncoderGet.vi"("EncoderDevRef"=w442) -> ("Distance"=w431:dbl, "EncoderDevRef"=w440:T8)  [unwired: 5 in, 4 out]
            n174 = call <vilib>:"WPI_EncoderGet.vi"("EncoderDevRef"=w441) -> ("Distance"=w438:dbl, "EncoderDevRef"=w439:T8)  [unwired: 5 in, 4 out]
            n175 = Unbundle By Name(w435) -> ("Yaw"=w434:dbl)
            n176 = Greater Or Equal?(x=w431, y=w430) -> (x >= y?=w429:bool)
            n177 = Greater Or Equal?(x=w438, y=w430) -> (x >= y?=w437:bool)
            n178 = Compound Arithmetic op=AND(w429, w437) -> (w436:bool)
            n179 = case shown="False" w436 {
              tunnel: w434 -> [w445 _]
              tunnel: w433 -> [w444 w466]
              tunnel: [w443 w465] -> w432
              frame False {
                n180 = Greater Or Equal?(x=w445, y=2.0) -> (x >= y?=w446:bool)
                n181 = case shown="True" w446 {
                  tunnel: w445 -> [_ w456]
                  tunnel: w444 -> [w449 w453]
                  tunnel: [w448 w452] -> w443
                  frame False {
                    n182 = call <vilib>:"WPI_RobotDriveTankDrive.vi"("Right axis value"=1.0, "Left axis value"=0.75, "RobotDriveDevRef"=w449) -> ("RobotDriveDevRef"=w448:T3)  [unwired: 6 in, 2 out]
                  }
                  frame True {
                    n183 = Less Or Equal?(x=w456, y=-2.0) -> (x <= y?=w454:bool)
                    n184 = case shown="False" w454 {
                      tunnel: w453 -> [w458 w461]
                      tunnel: [w457 w460] -> w452
                      frame False {
                        w459 = 1.0 ("Left axis value")
                        n185 = call <vilib>:"WPI_RobotDriveTankDrive.vi"("Right axis value"=w459, "Left axis value"=w459, "RobotDriveDevRef"=w458) -> ("RobotDriveDevRef"=w457:T3)  [unwired: 6 in, 2 out]
                      }
                      frame True {
                        n186 = call <vilib>:"WPI_RobotDriveTankDrive.vi"("Right axis value"=0.75, "Left axis value"=1.0, "RobotDriveDevRef"=w461) -> ("RobotDriveDevRef"=w460:T3)  [unwired: 6 in, 2 out]
                      }
                    }
                  }
                }
              }
              frame True {
                w467 = 0.0 ("Left axis value")
                n187 = global write "Robot Global Data.vi" "Enable Gear Tracking"(FALSE ("Enable Gear Tracking")) -> ()
                n188 = call <vilib>:"WPI_RobotDriveTankDrive.vi"("Right axis value"=w467, "Left axis value"=w467, "RobotDriveDevRef"=w466) -> ("RobotDriveDevRef"=w465:T3)  [unwired: 6 in, 2 out]
              }
            }
          }
        }
        frame #2 {
          n189 = Wait (ms)(milliseconds to wait=u32 10) -> ()  [unwired: 1 out]
          n190 = call-poly <vilib>:"WPI_SolenoidSet.vi"("Value"=WPI_SolenoidValue."Forward", "SolenoidDevRef"=w473) -> ("SolenoidDevRef"=w471:T12)  [unwired: 8 in, 1 out]
        }
        frame #3 {
          n191 = while {
            shift-right: [w485] -> _
            shift-left: w477 -> [w487]
            shift-right: [w486] -> _
            shift-left: w476 -> [w488]
            shift-right: [w481] -> w475
            shift-left: w478 -> [w492]
            stop <- w482 stop-if-true
            w490 = 48.0
            n192 = call <vilib>:"WPI_EncoderGet.vi"("EncoderDevRef"=w488) -> ("Distance"=w491:dbl, "EncoderDevRef"=w486:T8)  [unwired: 5 in, 4 out]
            n193 = call <vilib>:"WPI_EncoderGet.vi"("EncoderDevRef"=w487) -> ("Distance"=w489:dbl, "EncoderDevRef"=w485:T8)  [unwired: 5 in, 4 out]
            n194 = Less Or Equal?(x=w491, y=w490) -> (x <= y?=w484:bool)
            n195 = Less Or Equal?(x=w489, y=w490) -> (x <= y?=w483:bool)
            n196 = Compound Arithmetic op=AND(w484, w483) -> (w482:bool)
            n197 = case shown="True" w482 {
              tunnel: w492 -> [w496 w498]
              tunnel: [w493 w497] -> w481
              frame False {
                n198 = call <vilib>:"WPI_RobotDriveTankDrive.vi"("Right axis value"=-0.75, "Left axis value"=-0.75, "RobotDriveDevRef"=w496) -> ("RobotDriveDevRef"=w493:T3)  [unwired: 6 in, 2 out]
              }
              frame True {
                w499 = 0.0 ("Left axis value")
                n199 = call <vilib>:"WPI_RobotDriveTankDrive.vi"("Right axis value"=w499, "Left axis value"=w499, "RobotDriveDevRef"=w498) -> ("RobotDriveDevRef"=w497:T3)  [unwired: 6 in, 2 out]
              }
            }
          }
          n200 = call-poly <vilib>:"WPI_SolenoidSet.vi"("Value"=WPI_SolenoidValue."Reverse", "SolenoidDevRef"=w479) -> ()  [unwired: 8 in, 2 out]
        }
        frame #4 {
          n201 = while {
            shift-right: [w505] -> _
            shift-left: w500 -> [w506]
            stop <- w501 stop-if-true
            n202 = call <vilib>:"Get_YPRHfH.vi"() -> ("YRPHfH"=w510:T16)  [unwired: 11 in]
            n203 = Unbundle By Name(w510) -> ("Yaw"=w504:dbl)
            n204 = call-poly <vilib>:"PID.vi"("PID gains"=T15 {"proportional gain (Kc)"=1.0, "integral time (Ti, min)"=0.01, "derivative time (Td, min)"=0.0}, "process variable"=w504, "setpoint"=-60.0) -> ("output"=w507:dbl)  [unwired: 7 in, 1 out]
            n205 = In Range and Coerce(upper limit=-58.0, x=w504, lower limit=-62.0) -> (In Range?=w501:bool)  [unwired: 1 out]
            n206 = call <vilib>:"WPI_RobotDriveTankDrive.vi"("Left axis value"=w507, "RobotDriveDevRef"=w506) -> ("RobotDriveDevRef"=w505:T3)  [unwired: 7 in, 2 out]
          }
        }
        frame #5 {
        }
      }
    }
    frame "Right Gear Red" {
      n207 = flat-sequence {
        tunnel: w519 -> [w541]
        tunnel: w520 -> [w540]
        tunnel: w521 -> [w539]
        tunnel: [w535] -> w531
        tunnel: [w534] -> w530
        tunnel: [w533] -> w529
        tunnel: [w532] -> w528
        tunnel: w522 -> [w532]
        tunnel: w531 -> [w551]
        tunnel: w530 -> [w550]
        tunnel: w529 -> [w547]
        tunnel: [w546] -> w518
        tunnel: w528 -> [w546]
        tunnel: [w545] -> w516
        tunnel: [w544] -> w514
        tunnel: [w543] -> w512
        tunnel: w518 -> [w595]
        tunnel: [w595] -> w517
        tunnel: w516 -> [w594]
        tunnel: [w593] -> w515
        tunnel: w514 -> [w592]
        tunnel: [w592] -> w513
        tunnel: w512 -> [w591]
        tunnel: [w591] -> w511
        tunnel: w517 -> [w611]
        tunnel: [w609] -> w527
        tunnel: [w608] -> w526
        tunnel: w515 -> [w608]
        tunnel: [w607] -> w525
        tunnel: w513 -> [w607]
        tunnel: [w606] -> w524
        tunnel: w511 -> [w606]
        tunnel: w527 -> [w617]
        tunnel: w526 -> [w616]
        tunnel: w525 -> [w614]
        tunnel: w524 -> [w615]
        tunnel: [w613] -> w523
        tunnel: w523 -> [_]
        frame #0 {
          w538 = FALSE
          w542 = 0.0 ("Left axis value")
          n208 = call <vilib>:"Zero Yaw.vi"() -> ()  [unwired: 12 in]
          n209 = call <vilib>:"WPI_EncoderReset.vi"("EncoderDevRef"=w539) -> ("EncoderDevRef"=w534:T8)  [unwired: 9 in, 1 out]
          n210 = call <vilib>:"WPI_EncoderReset.vi"("EncoderDevRef"=w540) -> ("EncoderDevRef"=w535:T8)  [unwired: 9 in, 1 out]
          n211 = call <vilib>:"WPI_RobotDriveTankDrive.vi"("Right axis value"=w542, "Left axis value"=w542, "RobotDriveDevRef"=w541) -> ("RobotDriveDevRef"=w533:T3)  [unwired: 6 in, 2 out]
          n212 = global write "Robot Global Data.vi" "Enable Gear Tracking"(w538) -> ()
          n213 = global write "Robot Global Data.vi" "Center Gear"(TRUE ("Center Gear")) -> ()
          n214 = global write "Robot Global Data.vi" "Rev up"(w538) -> ()
          n215 = global write "Robot Global Data.vi" "Shoot"(w538) -> ()
          n216 = Wait (ms)(milliseconds to wait=u32 10) -> ()  [unwired: 1 out]
        }
        frame #1 {
          n217 = global write "Robot Global Data.vi" "Center Gear"(FALSE ("Center Gear")) -> ()
          n218 = global write "Robot Global Data.vi" "Enable Gear Tracking"(TRUE ("Enable Gear Tracking")) -> ()
          n219 = while {
            shift-right: [w563] -> w544
            shift-left: w551 -> [w565]
            shift-right: [w562] -> w543
            shift-left: w550 -> [w564]
            shift-right: [w555] -> w545
            shift-left: w547 -> [w556]
            stop <- w559 stop-if-true
            w553 = 68.0
            n220 = call <vilib>:"Get_YPRHfH.vi"() -> ("YRPHfH"=w558:T16)  [unwired: 11 in]
            n221 = call <vilib>:"WPI_EncoderGet.vi"("EncoderDevRef"=w565) -> ("Distance"=w554:dbl, "EncoderDevRef"=w563:T8)  [unwired: 5 in, 4 out]
            n222 = call <vilib>:"WPI_EncoderGet.vi"("EncoderDevRef"=w564) -> ("Distance"=w561:dbl, "EncoderDevRef"=w562:T8)  [unwired: 5 in, 4 out]
            n223 = Unbundle By Name(w558) -> ("Yaw"=w557:dbl)
            n224 = Greater Or Equal?(x=w554, y=w553) -> (x >= y?=w552:bool)
            n225 = Greater Or Equal?(x=w561, y=w553) -> (x >= y?=w560:bool)
            n226 = Compound Arithmetic op=AND(w552, w560) -> (w559:bool)
            n227 = case shown="False" w559 {
              tunnel: w557 -> [w568 _]
              tunnel: w556 -> [w567 w589]
              tunnel: [w566 w588] -> w555
              frame False {
                n228 = Greater Or Equal?(x=w568, y=2.0) -> (x >= y?=w569:bool)
                n229 = case shown="True" w569 {
                  tunnel: w568 -> [_ w579]
                  tunnel: w567 -> [w572 w576]
                  tunnel: [w571 w575] -> w566
                  frame False {
                    n230 = call <vilib>:"WPI_RobotDriveTankDrive.vi"("Right axis value"=1.0, "Left axis value"=0.75, "RobotDriveDevRef"=w572) -> ("RobotDriveDevRef"=w571:T3)  [unwired: 6 in, 2 out]
                  }
                  frame True {
                    n231 = Less Or Equal?(x=w579, y=-2.0) -> (x <= y?=w577:bool)
                    n232 = case shown="False" w577 {
                      tunnel: w576 -> [w581 w584]
                      tunnel: [w580 w583] -> w575
                      frame False {
                        w582 = 1.0 ("Left axis value")
                        n233 = call <vilib>:"WPI_RobotDriveTankDrive.vi"("Right axis value"=w582, "Left axis value"=w582, "RobotDriveDevRef"=w581) -> ("RobotDriveDevRef"=w580:T3)  [unwired: 6 in, 2 out]
                      }
                      frame True {
                        n234 = call <vilib>:"WPI_RobotDriveTankDrive.vi"("Right axis value"=0.75, "Left axis value"=1.0, "RobotDriveDevRef"=w584) -> ("RobotDriveDevRef"=w583:T3)  [unwired: 6 in, 2 out]
                      }
                    }
                  }
                }
              }
              frame True {
                w590 = 0.0 ("Left axis value")
                n235 = global write "Robot Global Data.vi" "Enable Gear Tracking"(FALSE ("Enable Gear Tracking")) -> ()
                n236 = call <vilib>:"WPI_RobotDriveTankDrive.vi"("Right axis value"=w590, "Left axis value"=w590, "RobotDriveDevRef"=w589) -> ("RobotDriveDevRef"=w588:T3)  [unwired: 6 in, 2 out]
              }
            }
          }
        }
        frame #2 {
          n237 = while {
            shift-right: [w600] -> w593
            shift-left: w594 -> [w601]
            stop <- w596 stop-if-true
            n238 = call <vilib>:"Get_YPRHfH.vi"() -> ("YRPHfH"=w605:T16)  [unwired: 11 in]
            n239 = Unbundle By Name(w605) -> ("Yaw"=w599:dbl)
            n240 = call-poly <vilib>:"PID.vi"("PID gains"=T15 {"proportional gain (Kc)"=1.0, "integral time (Ti, min)"=0.01, "derivative time (Td, min)"=0.0}, "process variable"=w599, "setpoint"=-45.0) -> ("output"=w602:dbl)  [unwired: 7 in, 1 out]
            n241 = In Range and Coerce(upper limit=-43.0, x=w599, lower limit=-47.0) -> (In Range?=w596:bool)  [unwired: 1 out]
            n242 = call <vilib>:"WPI_RobotDriveTankDrive.vi"("Left axis value"=w602, "RobotDriveDevRef"=w601) -> ("RobotDriveDevRef"=w600:T3)  [unwired: 7 in, 2 out]
          }
        }
        frame #3 {
          n243 = Wait (ms)(milliseconds to wait=u32 10) -> ()  [unwired: 1 out]
          n244 = call-poly <vilib>:"WPI_SolenoidSet.vi"("Value"=WPI_SolenoidValue."Forward", "SolenoidDevRef"=w611) -> ("SolenoidDevRef"=w609:T12)  [unwired: 8 in, 1 out]
        }
        frame #4 {
          n245 = while {
            shift-right: [w623] -> _
            shift-left: w615 -> [w625]
            shift-right: [w624] -> _
            shift-left: w614 -> [w626]
            shift-right: [w619] -> w613
            shift-left: w616 -> [w630]
            stop <- w620 stop-if-true
            w628 = 60.0
            n246 = call <vilib>:"WPI_EncoderGet.vi"("EncoderDevRef"=w626) -> ("Distance"=w629:dbl, "EncoderDevRef"=w624:T8)  [unwired: 5 in, 4 out]
            n247 = call <vilib>:"WPI_EncoderGet.vi"("EncoderDevRef"=w625) -> ("Distance"=w627:dbl, "EncoderDevRef"=w623:T8)  [unwired: 5 in, 4 out]
            n248 = Less Or Equal?(x=w629, y=w628) -> (x <= y?=w622:bool)
            n249 = Less Or Equal?(x=w627, y=w628) -> (x <= y?=w621:bool)
            n250 = Compound Arithmetic op=AND(w622, w621) -> (w620:bool)
            n251 = case shown="True" w620 {
              tunnel: w630 -> [w634 w636]
              tunnel: [w631 w635] -> w619
              frame False {
                n252 = call <vilib>:"WPI_RobotDriveTankDrive.vi"("Right axis value"=-0.75, "Left axis value"=-0.75, "RobotDriveDevRef"=w634) -> ("RobotDriveDevRef"=w631:T3)  [unwired: 6 in, 2 out]
              }
              frame True {
                w637 = 0.0 ("Left axis value")
                n253 = call <vilib>:"WPI_RobotDriveTankDrive.vi"("Right axis value"=w637, "Left axis value"=w637, "RobotDriveDevRef"=w636) -> ("RobotDriveDevRef"=w635:T3)  [unwired: 6 in, 2 out]
              }
            }
          }
          n254 = call-poly <vilib>:"WPI_SolenoidSet.vi"("Value"=WPI_SolenoidValue."Reverse", "SolenoidDevRef"=w617) -> ()  [unwired: 8 in, 2 out]
        }
        frame #5 {
        }
      }
    }
    frame "Left Gear Red" {
      n255 = flat-sequence {
        tunnel: w641 -> [w668]
        tunnel: w640 -> [w667]
        tunnel: w639 -> [w666]
        tunnel: [w662] -> w658
        tunnel: [w661] -> w657
        tunnel: [w660] -> w656
        tunnel: [w659] -> w655
        tunnel: w638 -> [w659]
        tunnel: w658 -> [w678]
        tunnel: w657 -> [w677]
        tunnel: w656 -> [w674]
        tunnel: [w673] -> w654
        tunnel: w655 -> [w673]
        tunnel: [w672] -> w653
        tunnel: [w671] -> w652
        tunnel: [w670] -> w651
        tunnel: w654 -> [w722]
        tunnel: [w722] -> w650
        tunnel: w653 -> [w721]
        tunnel: [w720] -> w649
        tunnel: w652 -> [w719]
        tunnel: [w719] -> w648
        tunnel: w651 -> [w718]
        tunnel: [w718] -> w647
        tunnel: w650 -> [w738]
        tunnel: [w736] -> w646
        tunnel: [w735] -> w645
        tunnel: w649 -> [w735]
        tunnel: [w734] -> w644
        tunnel: w648 -> [w734]
        tunnel: [w733] -> w643
        tunnel: w647 -> [w733]
        tunnel: w646 -> [w744]
        tunnel: w645 -> [w743]
        tunnel: w644 -> [w741]
        tunnel: w643 -> [w742]
        tunnel: [w740] -> w642
        tunnel: w642 -> [_]
        frame #0 {
          w665 = FALSE
          w669 = 0.0 ("Left axis value")
          n256 = call <vilib>:"Zero Yaw.vi"() -> ()  [unwired: 12 in]
          n257 = call <vilib>:"WPI_EncoderReset.vi"("EncoderDevRef"=w666) -> ("EncoderDevRef"=w661:T8)  [unwired: 9 in, 1 out]
          n258 = call <vilib>:"WPI_EncoderReset.vi"("EncoderDevRef"=w667) -> ("EncoderDevRef"=w662:T8)  [unwired: 9 in, 1 out]
          n259 = call <vilib>:"WPI_RobotDriveTankDrive.vi"("Right axis value"=w669, "Left axis value"=w669, "RobotDriveDevRef"=w668) -> ("RobotDriveDevRef"=w660:T3)  [unwired: 6 in, 2 out]
          n260 = global write "Robot Global Data.vi" "Enable Gear Tracking"(w665) -> ()
          n261 = global write "Robot Global Data.vi" "Center Gear"(TRUE ("Center Gear")) -> ()
          n262 = global write "Robot Global Data.vi" "Rev up"(w665) -> ()
          n263 = global write "Robot Global Data.vi" "Shoot"(w665) -> ()
          n264 = Wait (ms)(milliseconds to wait=u32 10) -> ()  [unwired: 1 out]
        }
        frame #1 {
          n265 = global write "Robot Global Data.vi" "Center Gear"(FALSE ("Center Gear")) -> ()
          n266 = global write "Robot Global Data.vi" "Enable Gear Tracking"(TRUE ("Enable Gear Tracking")) -> ()
          n267 = while {
            shift-right: [w690] -> w671
            shift-left: w678 -> [w692]
            shift-right: [w689] -> w670
            shift-left: w677 -> [w691]
            shift-right: [w682] -> w672
            shift-left: w674 -> [w683]
            stop <- w686 stop-if-true
            w680 = 68.0
            n268 = call <vilib>:"Get_YPRHfH.vi"() -> ("YRPHfH"=w685:T16)  [unwired: 11 in]
            n269 = call <vilib>:"WPI_EncoderGet.vi"("EncoderDevRef"=w692) -> ("Distance"=w681:dbl, "EncoderDevRef"=w690:T8)  [unwired: 5 in, 4 out]
            n270 = call <vilib>:"WPI_EncoderGet.vi"("EncoderDevRef"=w691) -> ("Distance"=w688:dbl, "EncoderDevRef"=w689:T8)  [unwired: 5 in, 4 out]
            n271 = Unbundle By Name(w685) -> ("Yaw"=w684:dbl)
            n272 = Greater Or Equal?(x=w681, y=w680) -> (x >= y?=w679:bool)
            n273 = Greater Or Equal?(x=w688, y=w680) -> (x >= y?=w687:bool)
            n274 = Compound Arithmetic op=AND(w679, w687) -> (w686:bool)
            n275 = case shown="False" w686 {
              tunnel: w684 -> [w695 _]
              tunnel: w683 -> [w694 w716]
              tunnel: [w693 w715] -> w682
              frame False {
                n276 = Greater Or Equal?(x=w695, y=2.0) -> (x >= y?=w696:bool)
                n277 = case shown="True" w696 {
                  tunnel: w695 -> [_ w706]
                  tunnel: w694 -> [w699 w703]
                  tunnel: [w698 w702] -> w693
                  frame False {
                    n278 = call <vilib>:"WPI_RobotDriveTankDrive.vi"("Right axis value"=1.0, "Left axis value"=0.75, "RobotDriveDevRef"=w699) -> ("RobotDriveDevRef"=w698:T3)  [unwired: 6 in, 2 out]
                  }
                  frame True {
                    n279 = Less Or Equal?(x=w706, y=-2.0) -> (x <= y?=w704:bool)
                    n280 = case shown="False" w704 {
                      tunnel: w703 -> [w708 w711]
                      tunnel: [w707 w710] -> w702
                      frame False {
                        w709 = 1.0 ("Left axis value")
                        n281 = call <vilib>:"WPI_RobotDriveTankDrive.vi"("Right axis value"=w709, "Left axis value"=w709, "RobotDriveDevRef"=w708) -> ("RobotDriveDevRef"=w707:T3)  [unwired: 6 in, 2 out]
                      }
                      frame True {
                        n282 = call <vilib>:"WPI_RobotDriveTankDrive.vi"("Right axis value"=0.75, "Left axis value"=1.0, "RobotDriveDevRef"=w711) -> ("RobotDriveDevRef"=w710:T3)  [unwired: 6 in, 2 out]
                      }
                    }
                  }
                }
              }
              frame True {
                w717 = 0.0 ("Left axis value")
                n283 = global write "Robot Global Data.vi" "Enable Gear Tracking"(FALSE ("Enable Gear Tracking")) -> ()
                n284 = call <vilib>:"WPI_RobotDriveTankDrive.vi"("Right axis value"=w717, "Left axis value"=w717, "RobotDriveDevRef"=w716) -> ("RobotDriveDevRef"=w715:T3)  [unwired: 6 in, 2 out]
              }
            }
          }
        }
        frame #2 {
          n285 = while {
            shift-right: [w727] -> w720
            shift-left: w721 -> [w728]
            stop <- w723 stop-if-true
            n286 = call <vilib>:"Get_YPRHfH.vi"() -> ("YRPHfH"=w732:T16)  [unwired: 11 in]
            n287 = Unbundle By Name(w732) -> ("Yaw"=w726:dbl)
            n288 = call-poly <vilib>:"PID.vi"("PID gains"=T15 {"proportional gain (Kc)"=1.0, "integral time (Ti, min)"=0.01, "derivative time (Td, min)"=0.0}, "process variable"=w726, "setpoint"=45.0) -> ("output"=w729:dbl)  [unwired: 7 in, 1 out]
            n289 = In Range and Coerce(upper limit=43.0, x=w726, lower limit=47.0) -> (In Range?=w723:bool)  [unwired: 1 out]
            n290 = call <vilib>:"WPI_RobotDriveTankDrive.vi"("Left axis value"=w729, "RobotDriveDevRef"=w728) -> ("RobotDriveDevRef"=w727:T3)  [unwired: 7 in, 2 out]
          }
        }
        frame #3 {
          n291 = Wait (ms)(milliseconds to wait=u32 10) -> ()  [unwired: 1 out]
          n292 = call-poly <vilib>:"WPI_SolenoidSet.vi"("Value"=WPI_SolenoidValue."Forward", "SolenoidDevRef"=w738) -> ("SolenoidDevRef"=w736:T12)  [unwired: 8 in, 1 out]
        }
        frame #4 {
          n293 = while {
            shift-right: [w750] -> _
            shift-left: w742 -> [w752]
            shift-right: [w751] -> _
            shift-left: w741 -> [w753]
            shift-right: [w746] -> w740
            shift-left: w743 -> [w757]
            stop <- w747 stop-if-true
            w755 = 60.0
            n294 = call <vilib>:"WPI_EncoderGet.vi"("EncoderDevRef"=w753) -> ("Distance"=w756:dbl, "EncoderDevRef"=w751:T8)  [unwired: 5 in, 4 out]
            n295 = call <vilib>:"WPI_EncoderGet.vi"("EncoderDevRef"=w752) -> ("Distance"=w754:dbl, "EncoderDevRef"=w750:T8)  [unwired: 5 in, 4 out]
            n296 = Less Or Equal?(x=w756, y=w755) -> (x <= y?=w749:bool)
            n297 = Less Or Equal?(x=w754, y=w755) -> (x <= y?=w748:bool)
            n298 = Compound Arithmetic op=AND(w749, w748) -> (w747:bool)
            n299 = case shown="True" w747 {
              tunnel: w757 -> [w761 w763]
              tunnel: [w758 w762] -> w746
              frame False {
                n300 = call <vilib>:"WPI_RobotDriveTankDrive.vi"("Right axis value"=-0.75, "Left axis value"=-0.75, "RobotDriveDevRef"=w761) -> ("RobotDriveDevRef"=w758:T3)  [unwired: 6 in, 2 out]
              }
              frame True {
                w764 = 0.0 ("Left axis value")
                n301 = call <vilib>:"WPI_RobotDriveTankDrive.vi"("Right axis value"=w764, "Left axis value"=w764, "RobotDriveDevRef"=w763) -> ("RobotDriveDevRef"=w762:T3)  [unwired: 6 in, 2 out]
              }
            }
          }
          n302 = call-poly <vilib>:"WPI_SolenoidSet.vi"("Value"=WPI_SolenoidValue."Reverse", "SolenoidDevRef"=w744) -> ()  [unwired: 8 in, 2 out]
        }
        frame #5 {
        }
      }
    }
  }
